vi "test.vi"() -> ()   [LabVIEW 2016]
panel:
  out "positioner status":T1
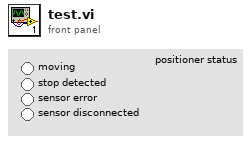
[diagram p1: front panel]
types:
  T1 = cluster{"moving":bool, "stop detected":bool, "sensor error":bool, "sensor disconnected":bool}
  T2 = cluster{"error ":bool, "error number":i32, "error code":string}
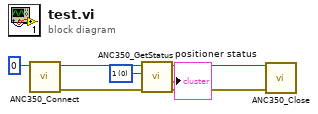
[diagram p0: block diagram]
diagram:
  w2 = u8 0 items=["1", "2", "3", "4", "5", "6", "7", "8", "9"] ("axis no")
  n1 = call "ANC350_Connect.vi"("device no"=0) -> ("error out"=w4:T2, "handle"=w6:i32)  [unwired: 5 in]
  n2 = call "ANC350_GetStatus.vi"("error in"=w4, "axis no"=w2, "device handle"=w6) -> ("error out"=w3:T2, "positioner status"=→"positioner status":T1, "device handle Out"=w5:i32)  [unwired: 2 in, 4 out]
  n3 = call "ANC350_Close.vi"("error in"=w3, "device handle"=w5) -> ()  [unwired: 5 in, 1 out]
